vi "Bairstow_Calculate bi&ci.vi"(0 "a(i)":dbl, 1 "s":dbl, 5 "b(i+1)":dbl, 7 "b(i+2)":dbl, 9 "c(i+1)":dbl, 11 "c(i+2)":dbl, 12 "r":dbl) -> (6 "b(i)":dbl, 15 "c(i)":dbl)   [LabVIEW 2020, in "NI_AALPro.lvlib"]
uses:
  NI_AALPro.lvlib
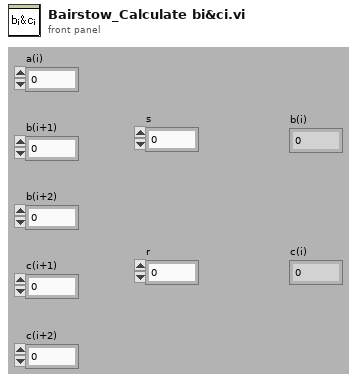
[diagram p1: front panel]
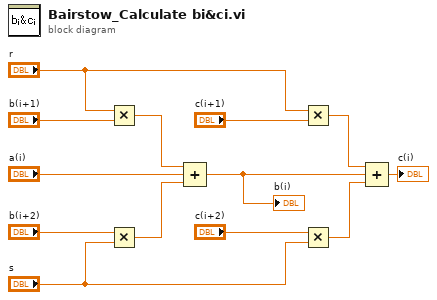
[diagram p0: block diagram]
diagram:
  n1 = Multiply(x="r", y="b(i+1)") -> (x*y=w10:dbl)
  n2 = Multiply(x="b(i+2)", y="s") -> (x*y=w11:dbl)
  n3 = Compound Arithmetic op=ADD(w10, "a(i)", w11) -> (w5:dbl)
  "b(i)" <- w5
  n4 = Multiply(x="r", y="c(i+1)") -> (x*y=w6:dbl)
  n5 = Multiply(x="c(i+2)", y="s") -> (x*y=w2:dbl)
  n6 = Compound Arithmetic op=ADD(w6, w5, w2) -> (→"c(i)":dbl)
